vi "DAQ_PW_RECORD_5000SP_calibrated.vi"(6 "waveform in":waveform(sgl), 9 "MA/UA":bool, 10 "calibration":dbl, 11 "DAQ in":refnum<k21>) -> (2 "waveform out 2":waveform(sgl), 3 "DAQ out":refnum<k21>)   [LabVIEW 2015]
uses:
  <vilib>/DAQmx/read.llb/DAQmx Read (Analog Wfm 1Chan NSamp).vi
  <vilib>/DAQmx/miscellaneous.llb/DAQmx Fill In Error Info.vi
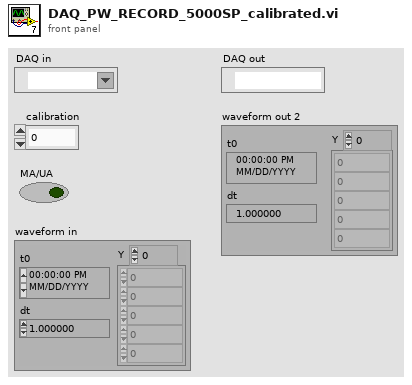
[diagram p1: front panel]
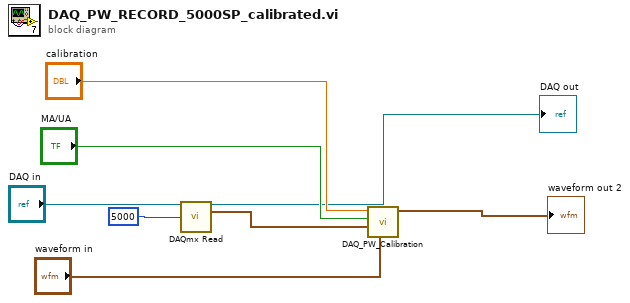
[diagram p0: block diagram]
diagram:
  n1 = call-poly <vilib>:"DAQmx Read.vi"("task/channels in"="DAQ in", "number of samples per channel"=5000) -> ("task out"=→"DAQ out":refnum<k21>, "data"=w7:waveform(dbl))  [unwired: 11 in, 1 out]
  n2 = call "DAQ_PW_Calibration.vi"("waveform in"="waveform in", "data"=w7, "MA/UA"="MA/UA", "calibration"="calibration") -> ("waveform out 2"=→"waveform out 2":waveform(sgl))  [unwired: 7 in]
